vi "Global Memory.vi"() -> ()   [LabVIEW 2021]
uses:
  Beam/Beam.lvclass
panel:
  in  "Mem":T1(c390)
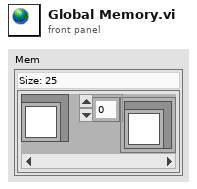
[diagram p1: front panel]
types:
  T1 = map{refnum<class "Beam.lvclass">, refnum<class "Beam.lvclass">[]}
diagram:
